vi "PyConv_CreateStructure.vi"(6 "UID":i32, 7 "PythonConverter_BD in":refnum<class "PyConvBD.lvclass">, 8 "error in":errorcluster, 11 "VI Interpreter in":refnum<class "VI Interpreter.lvclass">) -> (0 "error out":errorcluster, 3 "VI Interpreter out":refnum<class "VI Interpreter.lvclass">, 5 "PythonConverter_BD out":refnum<class "PyConvBD.lvclass">)   [LabVIEW 2014, in "PyConvBD.lvclass"]
uses:
  PyConvBD.lvclass
  VI Interpreter/Classes/VI Interpreter/VI Interpreter.lvclass
  VI Interpreter/Classes/Structure/Structure.lvclass
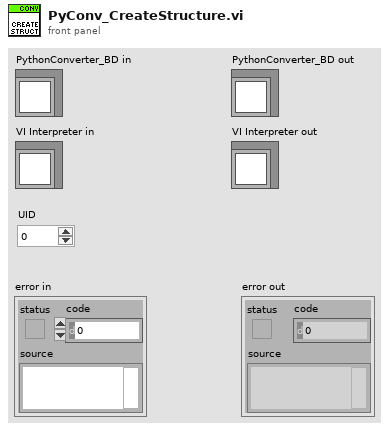
[diagram p1: front panel]
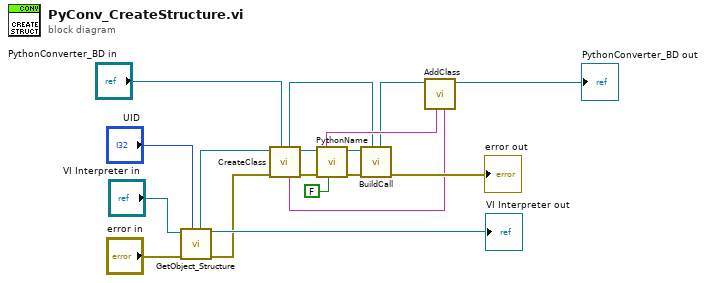
[diagram p0: block diagram]
diagram:
  n1 = call "GetObject_Structure.vi"("UID"="UID", "error in"="error in", "VI Interpreter in"="VI Interpreter in") -> ("error out"=w10:errorcluster, "VI Interpreter out"=→"VI Interpreter out":refnum<class "VI Interpreter.lvclass">, "structure"=w13:refnum<class "Structure.lvclass">)  [unwired: 3 in, 1 out]
  n2 = call-dynamic "CreateClass.vi"("PythonConverter_BD in"="PythonConverter_BD in", "error in"=w10, "GObject in"=w13) -> ("error out"=w16:errorcluster, "GObject out"=w17:refnum<class "Structure.lvclass">, "class"=w4:string, "PythonConverter_BD out"=w1:refnum<class "PyConvBD.lvclass">)  [unwired: 5 in]
  n3 = call-dynamic "PythonName.vi"("add self"=FALSE, "error in"=w16, "Node in"=w17) -> ("error out"=w8:errorcluster, "Node out"=w9:refnum<class "Structure.lvclass">, "UID"=w3:string)  [unwired: 5 in, 1 out]
  n4 = call-dynamic "BuildCall.vi"("PythonConverter_BD in"=w1, "error in"=w8, "Structure in"=w9) -> ("error out"=→"error out":errorcluster, "PythonConverter_BD out"=w2:refnum<class "PyConvBD.lvclass">)  [unwired: 6 in, 1 out]
  n5 = call "AddClass.vi"("definition"=w4, "name"=w3, "PythonConverter_BD in"=w2) -> ("PythonConverter_BD out"=→"PythonConverter_BD out":refnum<class "PyConvBD.lvclass">)  [unwired: 5 in, 1 out]
